vi "Global_HW_Data Out.vi"() -> ()   [LabVIEW 2017, in "Joystick.lvlib"]
uses:
  Joystick.lvlib
panel:
  in  "Sensor_HW_Int":i32
  in  "Sensor_HW_Bool":bool
  in  "Sensor_HW_DBL":dbl
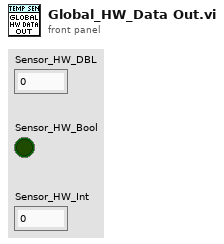
[diagram p1: front panel]
diagram:
